vi "test7-RegisterMultipleStatusesToOneState.vi"(8 "error in (no error)":errorcluster, 11 "TestCase in":refnum<class "testcase-CSMBroadcast.lvclass">) -> (0 "error out":errorcluster, 3 "TestCase out":refnum<class "testcase-CSMBroadcast.lvclass">)   [LabVIEW 2017, in "testcase-CSMBroadcast.lvclass"]
uses:
  testcase-CSMBroadcast.lvclass
  e86cc395-d992-44ca-a767-e0e34a6869d5.vi
  3bcad317-1b89-4687-aa9b-3ccbe7d60bbb.vi
  2694ea11-6498-4afa-8b48-991e2fec04f6.vi
  src/user.lib/_NEVSTOP/Communicable State Machine(CSM)/AdvanceAPI/CSM - Revert Arguments-Safe String.vi
  src/user.lib/_NEVSTOP/Communicable State Machine(CSM)/AdvanceAPI/CSM - Make String Arguments Safe.vi
  src/user.lib/_NEVSTOP/Communicable State Machine(CSM)/AdvanceAPI/CSM - Break Down Multiple States String.vi
  src/user.lib/_NEVSTOP/Communicable State Machine(CSM)/AdvanceAPI/CSM - Compact Multiple States.vi
  src/user.lib/_NEVSTOP/Communicable State Machine(CSM)/AdvanceAPI/CSM - Keywords.vi
  src/user.lib/_NEVSTOP/Communicable State Machine(CSM)/_Polymophic/CSM - Replace Marks in Messages.vi
  src/user.lib/_NEVSTOP/Communicable State Machine(CSM)/_Shared/Trim Single-line Text.vi
  src/user.lib/_NEVSTOP/Communicable State Machine(CSM)/AdvanceAPI/CSM - Set Module Attribute.vi
  src/user.lib/_NEVSTOP/Communicable State Machine(CSM)/AdvanceAPI/CSM - Get Module Attribute.vi
  <vilib>/addons/_JKI Toolkits/VI Tester/TestCase.llb/TestCase.lvclass
  src/user.lib/_NEVSTOP/Communicable State Machine(CSM)/Communicable State Machine.lvlib
  C:/Program Files (x86)/National Instruments/LabVIEW 2017/vi.lib/addons/_JKI Toolkits/VI Tester/TestCase.llb/TestCase.lvclass
panel:
  out "Error Out":errorcluster[](array[cluster])
  out "LoopCount":i32
  out "State History":string
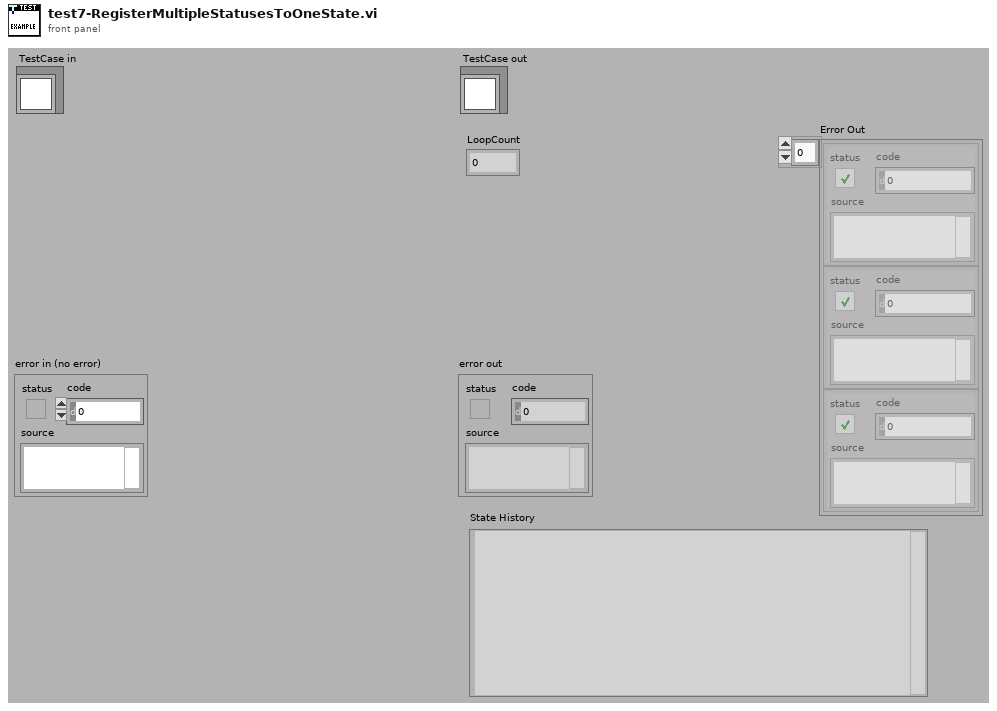
[diagram p1: front panel]
types:
  T1 = enum32{"Invalid", "Standard", "Closed", "Hidden", "Minimized", "Maximized"}
  T2 = enum32{"invalid app kind", "Development System", "Run Time System", "Student Edition", "Embedded LabVIEW", "Evaluation", "Custom"}
  T3 = typedef "Communicable State Machine.lvlib/_CSM_Response Source Message.ctl" = cluster{"‘State":string, "’Arguments":string, "’Error":errorcluster}
  T4 = cluster{"Current VI Reference":refnum<vi>, "Close Panel on Exit?":bool}
  T5 = cluster{"Core":cluster{"Current VI Reference":refnum<vi>, "Close Panel on Exit?":bool}, "Your Boolean data":bool, "Your string data":string, "TestData":i32}
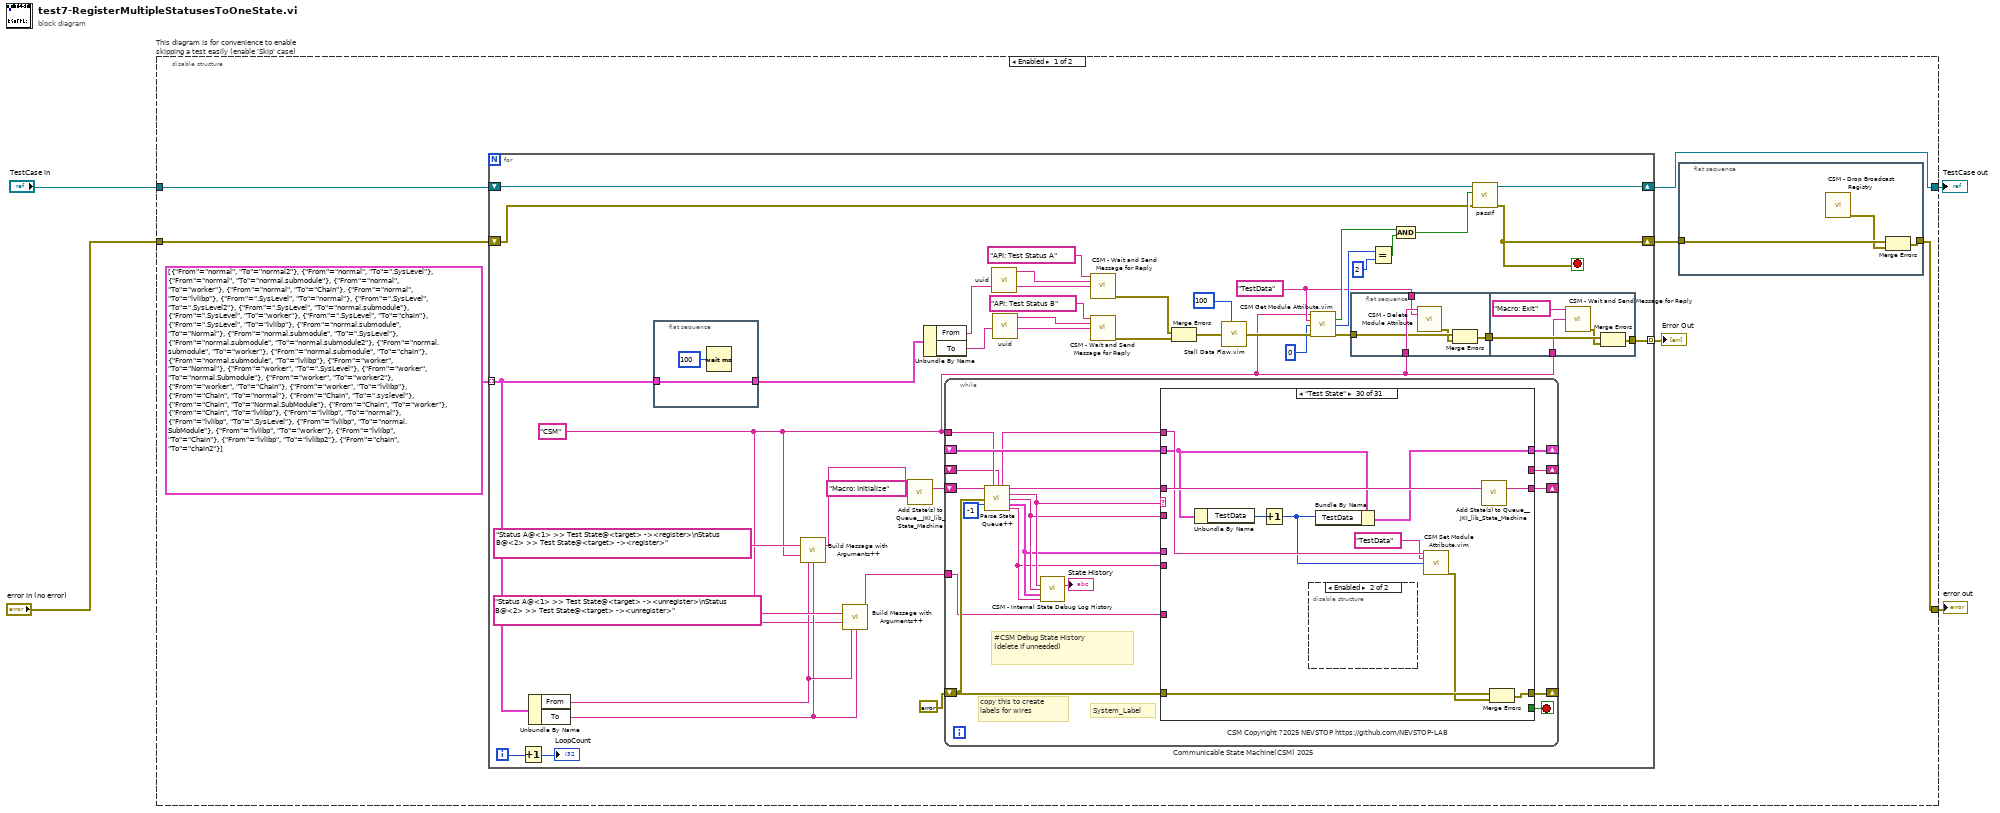
[diagram p0: block diagram]
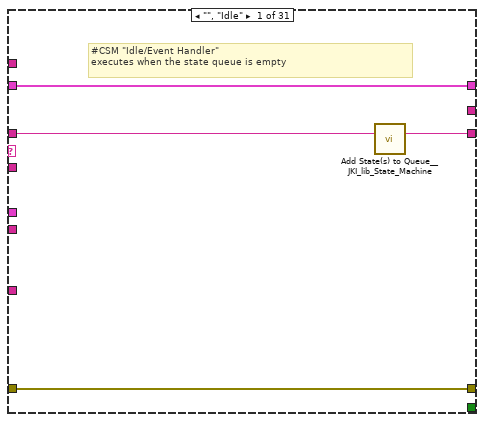
[diagram p2: hidden frame]
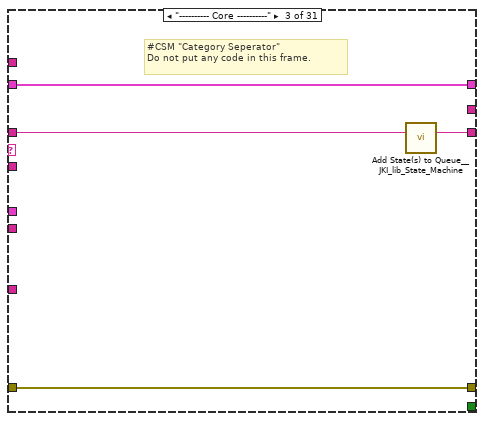
[diagram p4: hidden frame]
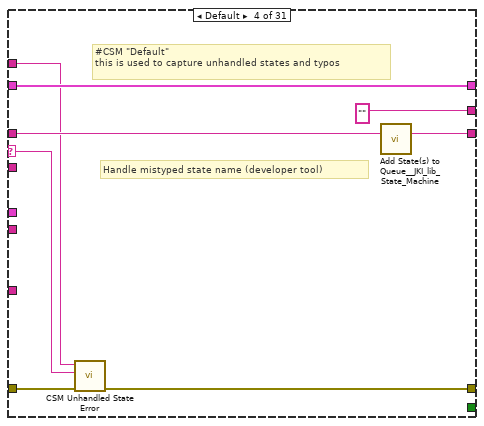
[diagram p5: hidden frame]
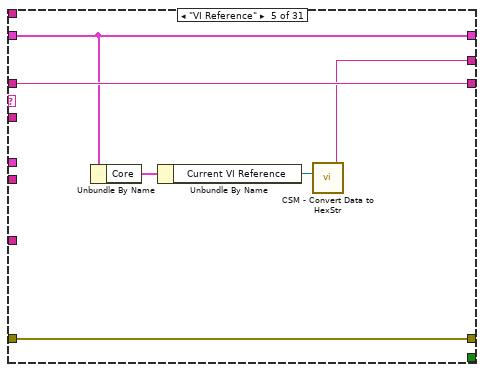
[diagram p6: hidden frame]
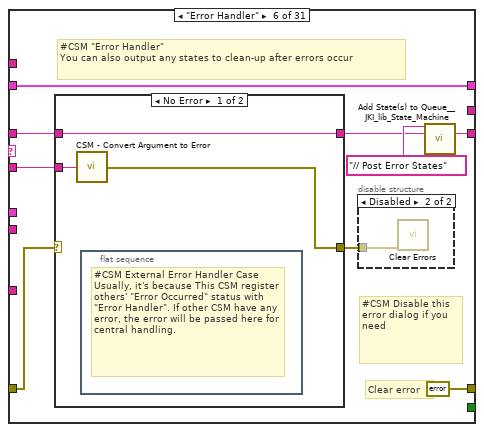
[diagram p7: hidden frame]
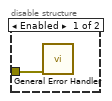
[diagram p8: hidden frame]
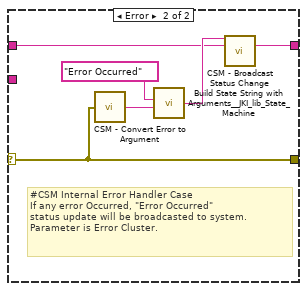
[diagram p9: hidden frame]
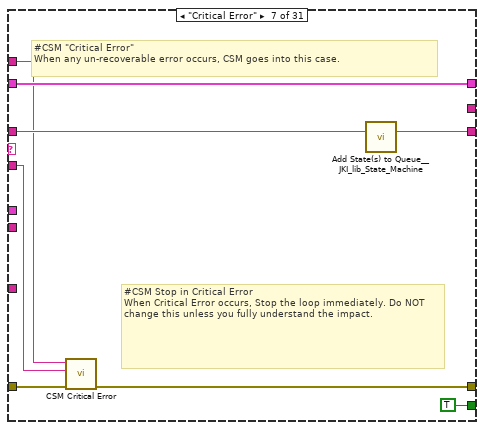
[diagram p10: hidden frame]
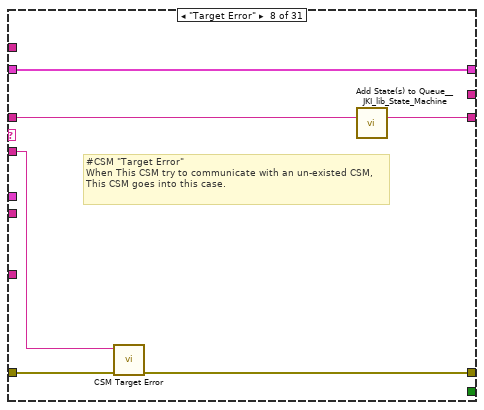
[diagram p11: hidden frame]
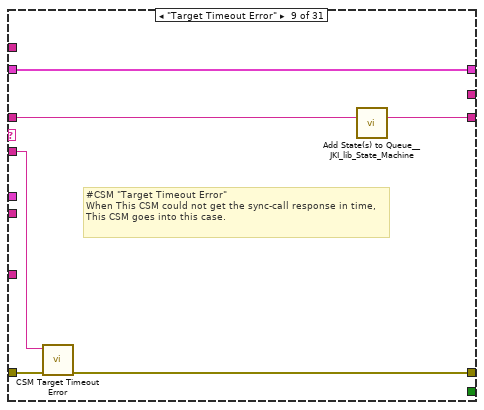
[diagram p12: hidden frame]
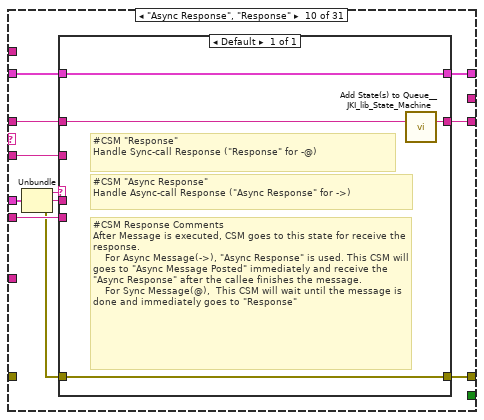
[diagram p13: hidden frame]
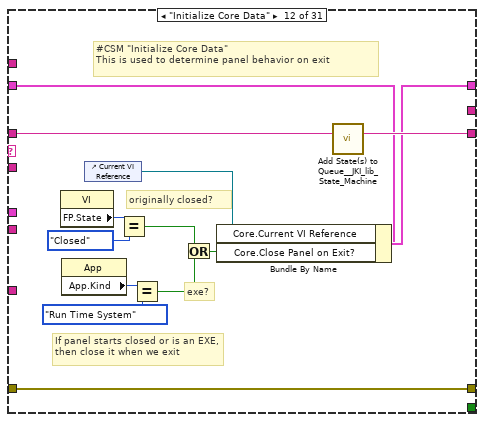
[diagram p15: hidden frame]
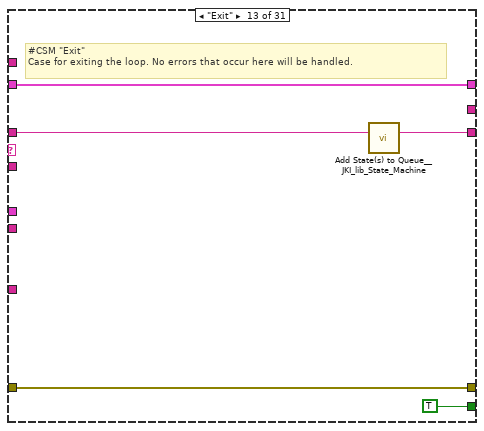
[diagram p16: hidden frame]
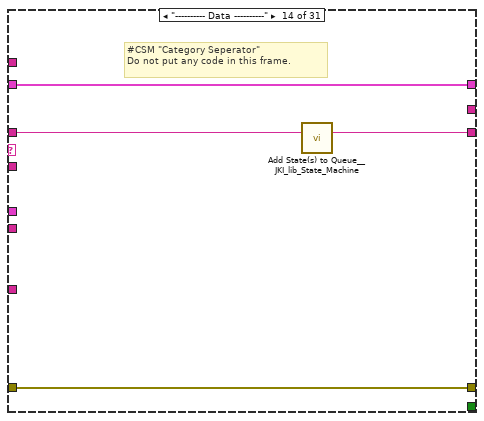
[diagram p17: hidden frame]
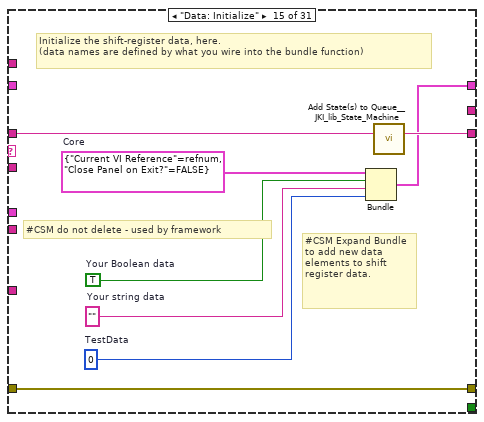
[diagram p18: hidden frame]
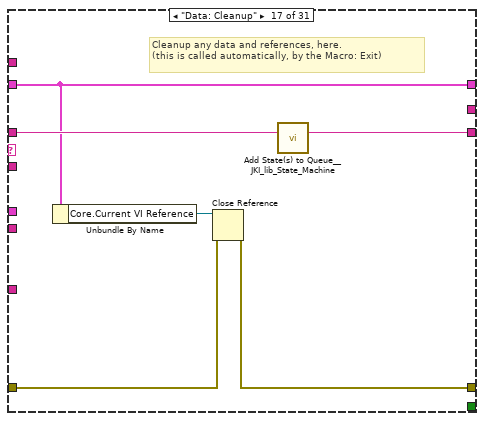
[diagram p20: hidden frame]
diagram:
  n1 = disable-structure "This diagram is for convenience to enable skipping a test easily (enable 'Skip' case)" shown="Enabled" {
    disable-tunnel: "TestCase in" -> [w10 w361]
    disable-tunnel: [w5 w359] -> w1
    disable-tunnel: [w6 w360] -> w3
    disable-tunnel: "error in (no error)" -> [w9 w358]
    frame Enabled {
      n2 = for {
        tunnel: cluster{"From":string, "To":string}[] [{"From"="normal", "To"="normal2"}, {"From"="normal", "To"=".SysLevel"}, {"From"="normal", "To"="normal.submodule"}, {"From"="normal", "To"="worker"}, {"From"="normal", "To"="Chain"}, {"From"="normal", "To"="lvlibp"}, {"From"=".SysLevel", "To"="normal"}, {"From"=".SysLevel", "To"=".SysLevel2"}, {"From"=".SysLevel", "To"="normal.submodule"}, {"From"=".SysLevel", "To"="worker"}, {"From"=".SysLevel", "To"="chain"}, {"From"=".SysLevel", "To"="lvlibp"}, {"From"="normal.submodule", "To"="Normal"}, {"From"="normal.submodule", "To"=".SysLevel"}, {"From"="normal.submodule", "To"="normal.submodule2"}, {"From"="normal.submodule", "To"="worker"}, {"From"="normal.submodule", "To"="chain"}, {"From"="normal.submodule", "To"="lvlibp"}, {"From"="worker", "To"="Normal"}, {"From"="worker", "To"=".SysLevel"}, {"From"="worker", "To"="normal.Submodule"}, {"From"="worker", "To"="worker2"}, {"From"="worker", "To"="Chain"}, {"From"="worker", "To"="lvlibp"}, {"From"="Chain", "To"="normal"}, {"From"="Chain", "To"=".syslevel"}, {"From"="Chain", "To"="Normal.SubModule"}, {"From"="Chain", "To"="worker"}, {"From"="Chain", "To"="lvlibp"}, {"From"="lvlibp", "To"="normal"}, {"From"="lvlibp", "To"=".SysLevel"}, {"From"="lvlibp", "To"="normal.SubModule"}, {"From"="lvlibp", "To"="worker"}, {"From"="lvlibp", "To"="Chain"}, {"From"="lvlibp", "To"="lvlibp2"}, {"From"="chain", "To"="chain2"}] -> [w42] mode=indexing
        shift-right: [w25] -> w5
        shift-left: w10 -> [w24]
        shift-right: [w22] -> w7
        shift-left: w9 -> [w23]
        tunnel: [w17] -> w8 mode=indexing
        i -> [w21]
        stop <- w22 stop-if-true
        w27 = "TestData" ("Attribute")
        w16 = "CSM" ("Name (\"\" to Use UUID)")
        n3 = Increment(x=w21) -> (x+1=→"LoopCount":i32)
        n4 = Unbundle By Name(w42) -> ("From"=w39:string, "To"=w38:string)
        n5 = flat-sequence {
          tunnel: w42 -> [w65]
          tunnel: [w65] -> w44
          frame #0 {
            n6 = Wait (ms)(milliseconds to wait=u32 100) -> ()  [unwired: 1 out]
          }
        }
        n7 = call-poly "Build Message with Arguments++.vi"("States With Replace Token"="Status A@<1> >> Test State@<target> -><register>\nStatus B@<2> >> Test State@<target> -><register>" ("Init State(\"Macro: Initialize\")"), "<target>"=w16, "<1>"=w39, "<2>"=w38) -> ("States"=w41:string)  [unwired: 11 in]
        n8 = call-poly "Build Message with Arguments++.vi"("States With Replace Token"="Status A@<1> >> Test State@<target> -><unregister>\nStatus B@<2> >> Test State@<target> -><unregister>" ("Init State(\"Macro: Initialize\")"), "<target>"=w16, "<1>"=w39, "<2>"=w38) -> ("States"=w37:string)  [unwired: 11 in]
        n9 = call <vilib>:"Add State(s) to Queue__JKI_lib_State_Machine.vi"("State(s) in Front (\"\")"=w41, "State(s) in (\"\")"="Macro: Initialize" ("Init State(\"Macro: Initialize\")")) -> ("States Out"=w45:string)  [unwired: 13 in]
        n10 = Unbundle By Name(w44) -> ("From"=w51:string, "To"=w50:string)
        n11 = while "Communicable State Machine(CSM) 2025" {
          shift-right: [w79] -> _
          shift-left: _ -> [w78]
          shift-right: [w82] -> _
          shift-left: errorcluster {"status"=FALSE, "code"=0, "source"=""} ("error out") -> [w77]
          shift-right: [w81] -> _
          shift-left: w45 -> [w83]
          tunnel: w16 -> [w75]
          shift-right: [w76] -> _
          shift-left: _ -> [w69]
          tunnel: w37 -> [w66]
          stop <- w80 stop-if-true
          # "#CSM Debug State History\n(delete if unneeded)"
          # "copy this to create labels for wires"
          # "System_Label"
          # "CSM Copyright ?2025 NEVSTOP https://github.com/NEVSTOP-LAB"
          n12 = call "Parse State Queue++.vi"("State Queue"=w83, "Name (\"\" to Use UUID)"=w75, "Response Arguments"=w69, "Previous Error"=w77, "Dequeue (1 ms)"=-1 ("Timeout")) -> ("Name Used"=w70:string, "Remaining States"=w84:string, "Current State"=w74:string, "Arguments"=w73:string, "Additional Information"=w72:T3, "Source CSM"=w71:string)  [unwired: 5 in]
          n13 = call "CSM - Internal State Debug Log History.vi"("State"=w74, "Arguments (\"\")"=w73, ">> Response Source Message >>"=w72, "Source (\"\")"=w71) -> ("Debug Log"=→"State History":string)  [unwired: 11 in]
          n14 = case shown="\"Test State\"" w74 {
            selector: w74 -> [_ _ _ w98 _ _ _ _ _ _ _ _ _ _ _ _ _ _ _ _ _ _ _ _ _ _ _ _ _ _ _]
            tunnel: w84 -> [w85 w90 w95 w102 w108 w114 w135 w141 w147 w155 w166 w180 w185 w189 w197 w199 w206 w210 w214 w220 w235 w304 w309 w317 w319 w323 w328 w335 w339 w350 w357]
            tunnel: w73 -> [_ _ _ _ _ w113 w131 w140 w145 w154 _ _ _ _ _ _ _ _ _ w215 w229 _ _ _ _ _ w326 _ _ _ _]
            tunnel: w78 -> [w86 w89 w92 w100 w107 w117 w136 w142 w148 w157 w165 w173 w183 w186 _ w198 w201 w207 w212 w218 w231 w301 w306 w314 w318 w322 w327 w332 w336 w342 w354]
            tunnel: [w87 w91 w93 w96 w109 errorcluster {"status"=FALSE, "code"=0, "source"=""} ("error out") w132 w138 w144 w160 w167 w177 w182 w187 w194 w200 w202 w208 w211 w216 w232 w302 w307 w315 w320 w324 w329 w333 w337 w344 w355] -> w82
            tunnel: w77 -> [w87 w91 w93 w103 w109 w115 w137 w139 w146 _ w167 w177 w182 w187 w194 w200 w203 w208 w211 w217 w233 w302 w307 w315 w320 w324 w329 w333 w337 w348 w355]
            tunnel: [w88 w90 w94 w101 w108 w110 w134 w143 w149 w156 w166 w179 w184 w188 w196 w199 w205 w209 w213 w219 w234 w303 w308 w316 w319 w323 w328 w334 w338 w349 w356] -> w81
            tunnel: [_ _ _ _ _ _ TRUE _ _ _ _ _ TRUE _ _ _ _ _ _ _ _ _ _ _ _ _ _ _ _ _ _] -> w80
            tunnel: [w86 w89 w92 w100 w107 w117 w136 w142 w148 w158 w165 w178 w183 w186 w195 w198 w201 w207 w212 w218 w231 w301 w306 w314 w318 w322 w327 w332 w336 w346 w354] -> w79
            tunnel: w71 -> [_ _ _ _ _ _ _ _ _ w152 _ _ _ _ _ _ _ _ _ _ _ _ _ _ _ _ _ _ _ _ _]
            tunnel: w72 -> [_ _ _ _ _ _ _ _ _ w159 _ _ _ _ _ _ _ _ _ _ _ _ _ _ _ _ _ _ _ _ _]
            tunnel: [_ _ _ "" w104 _ _ _ _ _ _ _ _ _ _ _ _ _ _ _ _ _ _ _ _ "API1 Response" w325 _ _ _ _] -> w76
            tunnel: w70 -> [_ _ _ w97 _ _ w130 _ _ _ _ _ _ _ _ _ _ _ _ _ _ _ _ _ _ _ _ _ _ w345 _]
            tunnel: w66 -> [_ _ _ _ _ _ _ _ _ _ _ _ _ _ _ _ _ _ _ _ _ _ _ w310 _ _ _ _ _ _ _]
            frame "", "Idle" {
              # "#CSM \"Idle/Event Handler\"\nexecutes when the state queue is empty"
              n15 = call <vilib>:"Add State(s) to Queue__JKI_lib_State_Machine.vi"("State(s) in (\"\")"=w85) -> ("States Out"=w88:string)  [unwired: 14 in]
            }
            frame "CSM Documentation" {
              # "#CSM README FIRST\n\nCommunicable State Machine(CSM) is a LabVIEW application framework that builds upon JKI State Machine(JKISM). It follows the pattern of JKISM and extends the keywords to describe message communication between modules, including concepts such as Sync-Message, Async-Message, Subscription/Unsubscription of status - essential elements for creating reusable code modules. For more information, please visit the CSM wiki: https://nevstop-lab.github.io/CSM-Wiki/\n\nFor instructions on JKI State Machine, visit: http://jki.net/state-machine/\nFor information about CSM, visit: https://github.com/NEVSTOP-LAB"
              # "#CSM \"Documentation\"\nCase for holding CSM Documenation"
            }
            frame "---------- Core ----------" {
              # "#CSM \"Category Seperator\"\nDo not put any code in this frame."
              n16 = call <vilib>:"Add State(s) to Queue__JKI_lib_State_Machine.vi"("State(s) in (\"\")"=w95) -> ("States Out"=w94:string)  [unwired: 14 in]
            }
            frame Default {
              # "#CSM \"Default\"\nthis is used to capture unhandled states and typos"
              # "Handle mistyped state name (developer tool)"
              n17 = call "CSM Unhandled State Error.vi"("error in (no error)"=w103, "Undefined State"=w98, "CSM Name"=w97) -> ("error out"=w96:errorcluster)  [unwired: 8 in]
              n18 = call <vilib>:"Add State(s) to Queue__JKI_lib_State_Machine.vi"("State(s) in (\"\")"=w102) -> ("States Out"=w101:string)  [unwired: 14 in]
            }
            frame "VI Reference" {
              n19 = Unbundle By Name(w107) -> ("Core"=w106:T4)
              n20 = Unbundle By Name(w106) -> ("Current VI Reference"=w105:refnum<vi>)
              n21 = call "CSM - Convert Data to HexStr.vi"("Variant"=w105) -> ("HEX String (0-9,A-F)"=w104:string)  [unwired: 8 in]
            }
            frame "Error Handler" {
              # "#CSM Disable this error dialog if you need"
              # "#CSM \"Error Handler\"\nYou can also output any states to clean-up after errors occur"
              # "Clear error"
              n22 = case shown="No Error" w115 {
                selector: w115 -> [_ w124]
                tunnel: [w123 w126] -> w111
                tunnel: w114 -> [w123 w125]
                tunnel: w113 -> [w122 _]
                tunnel: [w121 w124] -> w116
                frame No Error {
                  n23 = call "CSM - Convert Argument to Error.vi"("Argument"=w122) -> ("Error"=w121:errorcluster)  [unwired: 4 in]
                  n24 = flat-sequence {
                    frame #0 {
                      # "#CSM External Error Handler Case\nUsually, it's because This CSM register others' \"Error Occurred\" status with \"Error Handler\". If other CSM have any error, the error will be passed here for central handling."
                    }
                  }
                }
                frame Error {
                  # "#CSM Internal Error Handler Case \nIf any error Occurred, \"Error Occurred\" \nstatus update will be broadcasted to system.\nParameter is Error Cluster."
                  n25 = call "CSM - Convert Error to Argument.vi"("Error"=w124) -> ("Argument"=w128:string)  [unwired: 4 in]
                  n26 = call <vilib>:"Build State String with Arguments__JKI_lib_State_Machine.vi"("Arguments (\"\")"=w128, "State"="Error Occurred" ("Status with Arguments")) -> ("State with Arguments"=w127:string)  [unwired: 4 in]
                  n27 = call "CSM - Broadcast Status Change.vi"("Status With Arguments"=w127, "State Queue"=w125) -> ("Remaining States"=w126:string)  [unwired: 13 in]
                }
              }
              n28 = disable-structure shown="Disabled" {
                disable-tunnel: w116 -> [w119 w120]
                frame Enabled {
                  n29 = call <vilib>:"General Error Handler.vi"("error in (no error)"=w119) -> ()  [unwired: 10 in, 5 out]
                }
                frame Disabled {
                  n30 = call <vilib>:"Clear Errors.vi"("error in (no error)"=w120) -> ()  [unwired: 5 in, 2 out]
                }
              }
              n31 = call <vilib>:"Add State(s) to Queue__JKI_lib_State_Machine.vi"("State(s) in Front (\"\")"="// Post Error States", "State(s) in (\"\")"=w111) -> ("States Out"=w110:string)  [unwired: 13 in]
            }
            frame "Critical Error" {
              # "#CSM Stop in Critical Error\nWhen Critical Error occurs, Stop the loop immediately. Do NOT change this unless you fully understand the impact."
              # "#CSM \"Critical Error\"\nWhen any un-recoverable error occurs, CSM goes into this case."
              n32 = call "CSM Critical Error.vi"("error in (no error)"=w137, "Arugments (As Reason)"=w131, "CSM Name"=w130) -> ("error out"=w132:errorcluster)  [unwired: 8 in]
              n33 = call <vilib>:"Add State(s) to Queue__JKI_lib_State_Machine.vi"("State(s) in (\"\")"=w135) -> ("States Out"=w134:string)  [unwired: 14 in]
            }
            frame "Target Error" {
              # "#CSM \"Target Error\"\nWhen This CSM try to communicate with an un-existed CSM, This CSM goes into this case."
              n34 = call "CSM Target Error.vi"("error in (no error)"=w139, "Arguments (As CSM Name)"=w140) -> ("error out"=w138:errorcluster)  [unwired: 9 in]
              n35 = call <vilib>:"Add State(s) to Queue__JKI_lib_State_Machine.vi"("State(s) in (\"\")"=w141) -> ("States Out"=w143:string)  [unwired: 14 in]
            }
            frame "Target Timeout Error" {
              # "#CSM \"Target Timeout Error\"\nWhen This CSM could not get the sync-call response in time, This CSM goes into this case."
              n36 = call "CSM Target Timeout Error.vi"("error in (no error)"=w146, "Arguments (As CSM Name)"=w145) -> ("error out"=w144:errorcluster)  [unwired: 9 in]
              n37 = call <vilib>:"Add State(s) to Queue__JKI_lib_State_Machine.vi"("State(s) in (\"\")"=w147) -> ("States Out"=w149:string)  [unwired: 14 in]
            }
            frame "Async Response", "Response" {
              n38 = Unbundle(w159) -> ("‘State"=w153:string, "’Arguments"=w151:string, "’Error"=w150:errorcluster)
              n39 = case shown="Default" w153 {
                tunnel: [w164] -> w160
                tunnel: w150 -> [w164]
                tunnel: [w163] -> w158
                tunnel: w157 -> [w163]
                tunnel: [w161] -> w156
                tunnel: w155 -> [w162]
                tunnel: w154 -> [_]
                tunnel: w152 -> [_]
                tunnel: w151 -> [_]
                frame Default {
                  # "#CSM Response Comments\nAfter Message is executed, CSM goes to this state for receive the response.\n    For Async Message(->), \"Async Response\" is used. This CSM will goes to \"Async Message Posted\" immediately and receive the \"Async Response\" after the callee finishes the message.\n    For Sync Message(@),  This CSM will wait until the message is done and immediately goes to \"Response\""
                  # "#CSM \"Async Response\"\nHandle Async-call Response (\"Async Response\" for ->)"
                  # "#CSM \"Response\"\nHandle Sync-call Response (\"Response\" for -@)"
                  n40 = call <vilib>:"Add State(s) to Queue__JKI_lib_State_Machine.vi"("State(s) in (\"\")"=w162) -> ("States Out"=w161:string)  [unwired: 14 in]
                }
              }
            }
            frame "Async Message Posted" {
              # "#CSM \"Async Message Posted\"\nAfter Async Message is posted (-> or ->| ), CSM goes to this state for post-action.\nYou can use Argument - State to tell which Async Message is called."
            }
            frame "Initialize Core Data" {
              # "#CSM \"Initialize Core Data\"\nThis is used to determine panel behavior on exit"
              # "originally closed?"
              # "exe?"
              # "If panel starts closed or is an EXE, then close it when we exit"
              n41 = property class="VI"() -> ("FP.State"=w170:T1)  [unwired: 2 in, 2 out]
              n42 = property class="App"() -> ("App.Kind"=w176:T2)  [unwired: 2 in, 2 out]
              n43 = control-ref of="Current VI Reference"() -> (w171:refnum<vi>)
              n44 = Equal?(x=w170, y=T1."Closed" ("Front Panel Window:State")) -> (x = y?=w168:bool)
              n45 = Equal?(x=w176, y=T2."Run Time System" ("Application:Kind")) -> (x = y?=w174:bool)
              n46 = Or(x=w168, y=w174) -> (x .or. y?=w172:bool)
              n47 = Bundle By Name(cluster=w173, "Core.Current VI Reference"=w171, "Core.Close Panel on Exit?"=w172) -> (w178:T5)
              n48 = call <vilib>:"Add State(s) to Queue__JKI_lib_State_Machine.vi"("State(s) in (\"\")"=w180) -> ("States Out"=w179:string)  [unwired: 14 in]
            }
            frame "Exit" {
              # "#CSM \"Exit\"\nCase for exiting the loop. No errors that occur here will be handled."
              n49 = call <vilib>:"Add State(s) to Queue__JKI_lib_State_Machine.vi"("State(s) in (\"\")"=w185) -> ("States Out"=w184:string)  [unwired: 14 in]
            }
            frame "---------- Data ----------" {
              # "#CSM \"Category Seperator\"\nDo not put any code in this frame."
              n50 = call <vilib>:"Add State(s) to Queue__JKI_lib_State_Machine.vi"("State(s) in (\"\")"=w189) -> ("States Out"=w188:string)  [unwired: 14 in]
            }
            frame "Data: Initialize" {
              w190 = 0  # TestData
              w191 = T4 {"Current VI Reference"=refnum, "Close Panel on Exit?"=FALSE}  # Core
              w193 = TRUE  # Your Boolean data
              w192 = ""  # Your string data
              # "#CSM do not delete - used by framework"
              # "#CSM Expand Bundle to add new data elements to shift register data."
              # "Initialize the shift-register data, here.\n(data names are defined by what you wire into the bundle function)"
              n51 = Bundle("Core"=w191, "Your Boolean data"=w193, "Your string data"=w192, "TestData"=w190) -> (w195:T5)  [unwired: 1 in]
              n52 = call <vilib>:"Add State(s) to Queue__JKI_lib_State_Machine.vi"("State(s) in (\"\")"=w197) -> ("States Out"=w196:string)  [unwired: 14 in]
            }
            frame "Data: Update Indicators" {
            }
            frame "Data: Cleanup" {
              # "Cleanup any data and references, here.\n(this is called automatically, by the Macro: Exit)"
              n53 = Unbundle By Name(w201) -> ("Core.Current VI Reference"=w204:refnum<vi>)
              n54 = Close Reference(reference=w204, error in (no error)=w203) -> (error out=w202:errorcluster)
              n55 = call <vilib>:"Add State(s) to Queue__JKI_lib_State_Machine.vi"("State(s) in (\"\")"=w206) -> ("States Out"=w205:string)  [unwired: 14 in]
            }
            frame "---------- UI ----------" {
              # "#CSM \"Category Seperator\"\nDo not put any code in this frame."
              n56 = call <vilib>:"Add State(s) to Queue__JKI_lib_State_Machine.vi"("State(s) in (\"\")"=w210) -> ("States Out"=w209:string)  [unwired: 14 in]
            }
            frame "UI: Initialize" {
              # "#CSM \"UI: Initialize\"\nInitialize the User Interface, here.\n(this is called automatically, by the Macro: Init)"
              n57 = call <vilib>:"Add State(s) to Queue__JKI_lib_State_Machine.vi"("State(s) in (\"\")"=w214) -> ("States Out"=w213:string)  [unwired: 14 in]
            }
            frame "UI: Cursor Set" {
              # "#CSM \"UI: Cursor Set\"\nSet and Unset Cursor Busy.\n(Usage: \"UI: Cursor Set >> Busy|Idle\")"
              # "Argument"
              n58 = disable-structure shown="TARGET_TYPE!=Windows" {
                disable-tunnel: w217 -> [w223 w228]
                disable-tunnel: [w222 w228] -> w216
                disable-tunnel: w215 -> [w221 _]
                frame condition #0 (active) {
                  n59 = case shown="\"Idle\", Default" w221 {
                    tunnel: w223 -> [w225 w227]
                    tunnel: [w224 w226] -> w222
                    frame "Idle", Default {
                      n60 = call <vilib>:"Unset Busy.vi"("error in (no error)"=w225) -> ("error out"=w224:errorcluster)  [unwired: 10 in]
                    }
                    frame "Busy" {
                      n61 = call <vilib>:"Set Busy.vi"("error in (no error)"=w227) -> ("error out"=w226:errorcluster)  [unwired: 9 in, 1 out]
                    }
                  }
                }
                frame condition #1 {
                }
              }
              n62 = call <vilib>:"Add State(s) to Queue__JKI_lib_State_Machine.vi"("State(s) in (\"\")"=w220) -> ("States Out"=w219:string)  [unwired: 14 in]
            }
            frame "UI: Front Panel State" {
              # "#CSM \"UI: Front Panel State\"\nSet Front Panel Open or Closed\n(Usage: \"UI: Front Panel State >> Open|Close\")"
              # "Argument"
              n63 = Unbundle By Name(w231) -> ("Core.Current VI Reference"=w230:refnum<vi>)
              n64 = call <vilib>:"Add State(s) to Queue__JKI_lib_State_Machine.vi"("State(s) in (\"\")"=w235) -> ("States Out"=w234:string)  [unwired: 14 in]
              n65 = case shown="\"Close\", \"Closed\"" w229 {
                tunnel: w233 -> [w241 w256 w267 w280 w293]
                tunnel: [w243 w257 w269 w282 w295] -> w232
                tunnel: w230 -> [w242 w254 w268 w281 w294]
                frame "Open", "Standard", Default {
                  w236 = T1."Standard" ("State")
                  n66 = property class="VI"(reference=w242, error in=w241) -> (reference out=w239:refnum<vi>, error out=w240:errorcluster, "FP.State"=w238:T1)
                  n67 = Not Equal?(x=w238, y=w236) -> (x != y?=w237:bool)
                  n68 = case shown="True" w237 {
                    tunnel: [w247 w249] -> w243
                    tunnel: w240 -> [w246 w249]
                    tunnel: w239 -> [w245 _]
                    tunnel: w236 -> [w244 _]
                    frame True {
                      n69 = invoke class="VI" method="FP.Open"(reference=w245, error in=w246, "Activate"=TRUE, "State"=w244) -> (error out=w247:errorcluster)  [unwired: 1 in, 4 out]
                    }
                    frame False {
                    }
                  }
                }
                frame "Close", "Closed" {
                  n70 = property class="VI"(reference=w254, error in=w256) -> (reference out=w253:refnum<vi>, error out=w255:errorcluster, "FP.State"=w251:T1)
                  n71 = Not Equal?(x=w251, y=T1."Closed" ("Front Panel Window:State")) -> (x != y?=w250:bool)
                  n72 = case shown="False" w250 {
                    tunnel: [w258 w261] -> w257
                    tunnel: w255 -> [w258 w260]
                    tunnel: w253 -> [_ w259]
                    frame False {
                    }
                    frame True {
                      n73 = invoke class="VI" method="FP.Close"(reference=w259, error in=w260) -> (error out=w261:errorcluster)  [unwired: 1 in, 2 out]
                    }
                  }
                }
                frame "Hidden", "Hide" {
                  w262 = T1."Hidden" ("State")
                  n74 = property class="VI"(reference=w268, error in=w267) -> (reference out=w265:refnum<vi>, error out=w266:errorcluster, "FP.State"=w264:T1)
                  n75 = Not Equal?(x=w264, y=w262) -> (x != y?=w263:bool)
                  n76 = case shown="True" w263 {
                    tunnel: [w273 w274] -> w269
                    tunnel: w266 -> [w272 w274]
                    tunnel: w265 -> [w271 _]
                    tunnel: w262 -> [w270 _]
                    frame True {
                      n77 = invoke class="VI" method="FP.Open"(reference=w271, error in=w272, "State"=w270) -> (error out=w273:errorcluster)  [unwired: 2 in, 4 out]
                    }
                    frame False {
                    }
                  }
                }
                frame "Minimize", "Minimized" {
                  w275 = T1."Minimized" ("State")
                  n78 = property class="VI"(reference=w281, error in=w280) -> (reference out=w278:refnum<vi>, error out=w279:errorcluster, "FP.State"=w277:T1)
                  n79 = Not Equal?(x=w277, y=w275) -> (x != y?=w276:bool)
                  n80 = case shown="True" w276 {
                    tunnel: [w286 w287] -> w282
                    tunnel: w279 -> [w285 w287]
                    tunnel: w278 -> [w284 _]
                    tunnel: w275 -> [w283 _]
                    frame True {
                      n81 = invoke class="VI" method="FP.Open"(reference=w284, error in=w285, "State"=w283) -> (error out=w286:errorcluster)  [unwired: 2 in, 4 out]
                    }
                    frame False {
                    }
                  }
                }
                frame "Maximize", "Maximized" {
                  w288 = T1."Maximized" ("State")
                  n82 = property class="VI"(reference=w294, error in=w293) -> (reference out=w291:refnum<vi>, error out=w292:errorcluster, "FP.State"=w290:T1)
                  n83 = Not Equal?(x=w290, y=w288) -> (x != y?=w289:bool)
                  n84 = case shown="True" w289 {
                    tunnel: [w299 w300] -> w295
                    tunnel: w292 -> [w298 w300]
                    tunnel: w291 -> [w297 _]
                    tunnel: w288 -> [w296 _]
                    frame True {
                      n85 = invoke class="VI" method="FP.Open"(reference=w297, error in=w298, "State"=w296) -> (error out=w299:errorcluster)  [unwired: 2 in, 4 out]
                    }
                    frame False {
                    }
                  }
                }
              }
            }
            frame "---------- Macro ----------" {
              # "#CSM \"Category Seperator\"\nDo not put any code in this frame."
              n86 = call <vilib>:"Add State(s) to Queue__JKI_lib_State_Machine.vi"("State(s) in (\"\")"=w304) -> ("States Out"=w303:string)  [unwired: 14 in]
            }
            frame "Macro: Initialize" {
              # "#CSM \"Macro: Initialize\"\nInitialization Macro (This is called once, when the VI starts)"
              n87 = call <vilib>:"Add State(s) to Queue__JKI_lib_State_Machine.vi"("State(s) in Front (\"\")"="Data: Initialize\nInitialize Core Data\nData: Update Indicators", "State(s) in (\"\")"=w309) -> ("States Out"=w308:string)  [unwired: 13 in]
            }
            frame "Macro: Exit" {
              # "#CSM \"Macro: Exit\"\nExit Macro (This is called once, when the VI exits)"
              n88 = call <vilib>:"Add State(s) to Queue__JKI_lib_State_Machine.vi"("State(s) in Front (\"\")"="//Exit Sub-Modules ", "State(s) in (\"\")"=w310, "State(s) at Back (\"\")"="Data: Cleanup\nExit") -> ("States Out"=w312:string)  [unwired: 12 in]
              n89 = call <vilib>:"Add State(s) to Queue__JKI_lib_State_Machine.vi"("State(s) in Front (\"\")"=w312, "State(s) in (\"\")"=w317) -> ("States Out"=w316:string)  [unwired: 13 in]
            }
            frame "---------- API ----------" {
              # "#CSM \"Category Seperator\"\nDo not put any code in this frame."
            }
            frame "API: API1" {
              # "#CSM API Example\nCopy/Rename this case for your own API"
              # "#CSM Response\nConnect this to return the response of your API"
              # "#CSM >> Msg/Rep's CSM >>\nIf you need to tell who triggered this state , use this string. If it's this case itself, this string is \"\"."
              # "#CSM >> Arguments >>\nDeal with the parameter if any"
            }
            frame "API: API2" {
              # "#CSM API Example\nCopy/Rename this case for your own API"
              # "unpack Hex String  to Variant\nif complex parameter is needed."
              n90 = call "CSM - Convert HexStr to Data.vi"("HEX String"=w326) -> ()  [unwired: 7 in, 2 out]
              n91 = disable-structure shown="Disabled" {
                disable-tunnel: [w330 "API2 Response"] -> w325
                frame Disabled {
                  # "pack variant to hexstr \nif complex response is needed."
                  # "complex Response"
                  n92 = call "CSM - Convert Data to HexStr.vi"() -> ("HEX String (0-9,A-F)"=w330:string)  [unwired: 9 in]
                }
                frame Enabled {
                }
              }
            }
            frame "---------- Action ----------" {
              # "#CSM \"Category Seperator\"\nDo not put any code in this frame."
              n93 = call <vilib>:"Add State(s) to Queue__JKI_lib_State_Machine.vi"("State(s) in (\"\")"=w335) -> ("States Out"=w334:string)  [unwired: 14 in]
            }
            frame "Action: action1" {
              # "#CSM \"Internal State\"\nThis category is used for holding internal states"
              n94 = call <vilib>:"Add State(s) to Queue__JKI_lib_State_Machine.vi"("State(s) in (\"\")"=w339) -> ("States Out"=w338:string)  [unwired: 14 in]
            }
            frame "Test State" {
              n95 = Unbundle By Name(w342) -> ("TestData"=w347:i32)
              n96 = Increment(x=w347) -> (x+1=w340:i32)
              n97 = disable-structure shown="Enabled" {
                frame Disabled {
                  n98 = feedback #1(0 ("y")) -> (w352:i32)
                  n99 = Increment(x=w352) -> (x+1=w351:i32)
                  n100 = feedback-in #1(w351) -> ()
                }
                frame Enabled {
                }
              }
              n101 = Bundle By Name(cluster=w342, "TestData"=w340) -> (w346:T5)
              n102 = call "CSM Set Module Attribute.vim"("CSM Name"=w345, "Attribute"="TestData", "Value"=w340) -> ("error out"=w343:errorcluster)  [unwired: 9 in, 3 out]
              n103 = call <vilib>:"Add State(s) to Queue__JKI_lib_State_Machine.vi"("State(s) in (\"\")"=w350) -> ("States Out"=w349:string)  [unwired: 14 in]
              n104 = Merge Errors(w348, w343) -> (w344:errorcluster)
            }
            frame "Action: action2" {
              # "#CSM \"Internal State\"\nThis category is used for holding internal states"
              n105 = call <vilib>:"Add State(s) to Queue__JKI_lib_State_Machine.vi"("State(s) in (\"\")"=w357) -> ("States Out"=w356:string)  [unwired: 14 in]
            }
          }
        }
        n106 = call "uuid.vi"() -> ("UUID"=w49:string)  [unwired: 11 in]
        n107 = call "uuid.vi"() -> ("UUID"=w48:string)  [unwired: 11 in]
        n108 = call "CSM - Wait and Send Message for Reply.vi"("State"="API: Test Status A", "Arguments (\"\")"=w49, "Target Module"=w51) -> ("error out"=w36:errorcluster)  [unwired: 9 in, 3 out]
        n109 = call "CSM - Wait and Send Message for Reply.vi"("State"="API: Test Status B", "Arguments (\"\")"=w48, "Target Module"=w50) -> ("error out"=w35:errorcluster)  [unwired: 9 in, 3 out]
        n110 = Merge Errors(w36, w35) -> (w34:errorcluster)
        n111 = call "Stall Data Flow.vim"("value in"=w34, "milliseconds to wait"=u32 100) -> ("value out"=w32:errorcluster)  [unwired: 1 out]
        n112 = call "CSM Get Module Attribute.vim"("CSM Name"=w16, "Attribute"=w27, "Default Value (Empty Variant)"=0 ("y"), "Error In"=w32) -> ("Found"=w31:bool, "Value"=w30:i32, "error out"=w19:errorcluster)  [unwired: 7 in, 2 out]
        n113 = flat-sequence {
          tunnel: w16 -> [w58]
          tunnel: w27 -> [w57]
          tunnel: w19 -> [w56]
          tunnel: [w54] -> w18
          tunnel: w18 -> [w63]
          tunnel: [w61] -> w17
          tunnel: w16 -> [w59]
          frame #0 {
            n114 = call "CSM - Delete Module Attribute.vi"("CSM Name"=w58, "Attribute"=w57) -> ("error out"=w55:errorcluster)  [unwired: 10 in, 3 out]
            n115 = Merge Errors(w56, w55) -> (w54:errorcluster)
          }
          frame #1 {
            n116 = call "CSM - Wait and Send Message for Reply.vi"("State"="Macro: Exit", "Target Module"=w59) -> ("error out"=w62:errorcluster)  [unwired: 10 in, 3 out]
            n117 = Merge Errors(w63, w62) -> (w61:errorcluster)
          }
        }
        n118 = Equal?(x=w30, y=2) -> (x = y?=w28:bool)
        n119 = And(x=w31, y=w28) -> (x .and. y?=w26:bool)
        n120 = call-dynamic "passIf.vi"("error in (no error)"=w23, "pass"=w26, "TestCase in"=w24) -> ("error out"=w22:errorcluster, "TestCase out"=w25:refnum<class "testcase-CSMBroadcast.lvclass">)  [unwired: 7 in]
      }
      "Error Out" <- w8
      n121 = flat-sequence {
        tunnel: w7 -> [w14]
        tunnel: [w13] -> w6
        frame #0 {
          n122 = call "CSM - Drop Broadcast Registry.vi"() -> ("error out"=w12:errorcluster)  [unwired: 15 in]
          n123 = Merge Errors(w14, w12) -> (w13:errorcluster)
        }
      }
    }
    frame Disabled {
      # "skip test result while test is under development"
      n124 = call <vilib>:"skip.vi"("error in (no error)"=w358, "TestCase in"=w361) -> ("error out"=w360:errorcluster, "TestCase out"=w359:refnum<class "testcase-CSMBroadcast.lvclass">)  [unwired: 8 in]
    }
  }
  "error out" <- w3
  "TestCase out" <- w1
